vi "Write timeouts.vi"(8 "error in (no error)":errorcluster, 10 "timeouts":T1={"connect timeout"=60000, "write timeout"=10000, "read timeout"=10000}, 11 "TCP Master in":refnum<class "TCP.lvclass">) -> (0 "error out":errorcluster, 3 "TCP Master out":refnum<class "TCP.lvclass">)   [LabVIEW 2021, in "TCP.lvclass"]
uses:
  TCP.lvclass
  tcp timeouts.ctl
  TCP.lvclass/TCP.ctl
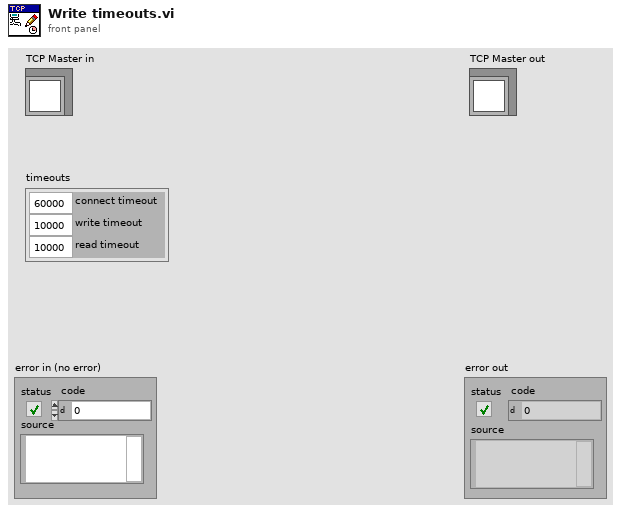
[diagram p1: front panel]
types:
  T1 = typedef "TCP.lvclass/tcp timeouts.ctl" = cluster{"connect timeout":i32, "write timeout":i32, "read timeout":i32}
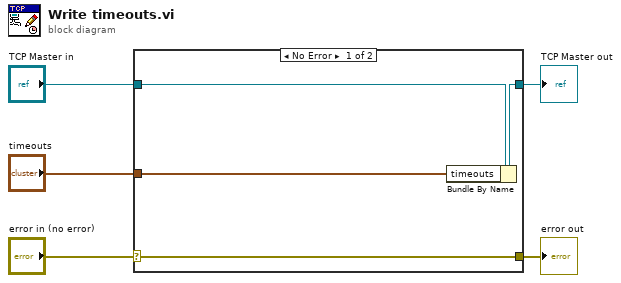
[diagram p0: block diagram]
diagram:
  n1 = case shown="No Error" "error in (no error)" {
    selector: "error in (no error)" -> [w9 w10]
    tunnel: [w9 w10] -> w4
    tunnel: [w7 w11] -> w2
    tunnel: "TCP Master in" -> [w8 w11]
    tunnel: "timeouts" -> [w6 _]
    frame No Error {
      n2 = Bundle By Name(cluster=w8, "timeouts"=w6) -> (w7:refnum<class "TCP.lvclass">)
    }
    frame Error {
    }
  }
  "error out" <- w4
  "TCP Master out" <- w2
